vi "Write Line.vi"(8 "error in (no error)":errorcluster, 10 "Line":i32, 11 "Set Output Line Msg in":refnum<class "Set Output Line Msg.lvclass">) -> (0 "error out":errorcluster, 3 "Set Output Line Msg out":refnum<class "Set Output Line Msg.lvclass">)   [LabVIEW 2020, in "BNT_ULx.lvlib" / "Set Output Line Msg.lvclass"]
uses:
  Set Output Line Msg.lvclass
  Set Output Line Msg.lvclass/Set Output Line Msg.ctl
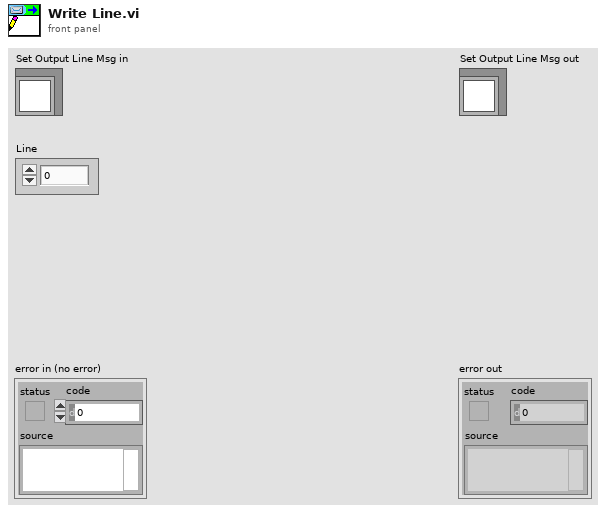
[diagram p1: front panel]
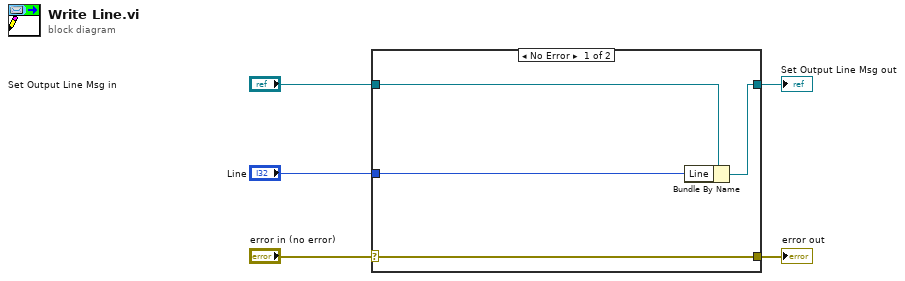
[diagram p0: block diagram]
diagram:
  n1 = case shown="No Error" "error in (no error)" {
    selector: "error in (no error)" -> [w9 w10]
    tunnel: [w9 w10] -> w4
    tunnel: [w7 w11] -> w2
    tunnel: "Set Output Line Msg in" -> [w8 w11]
    tunnel: "Line" -> [w6 _]
    frame No Error {
      n2 = Bundle By Name(cluster=w8, "Line"=w6) -> (w7:refnum<class "Set Output Line Msg.lvclass">)
    }
    frame Error {
    }
  }
  "error out" <- w4
  "Set Output Line Msg out" <- w2
